vi "SpectroMeterConnectCheck.vi"(0 "error in":errorcluster) -> (1 "error Out":errorcluster caption="error out", 2 "LightField Automation out":refnum<class "LightField Automation.lvclass">)   [LabVIEW 2018]
uses:
  C:/ProgramData/Documents/Princeton Instruments/LightField/Add-in and Automation SDK/Samples/LabVIEW Automation/lightfield-automation-labview/LightField Automation.lvclass
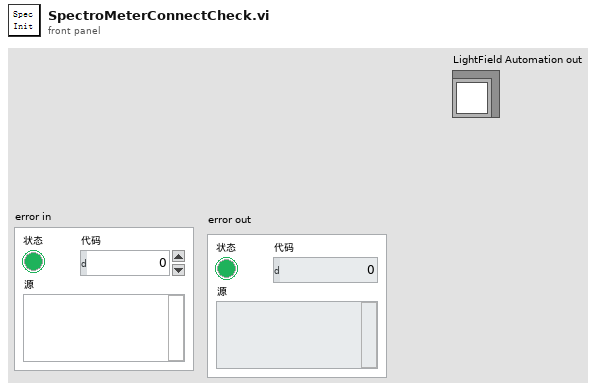
[diagram p1: front panel]
types:
  T1 = typedef "IMAQ Image.ctl" = refnum<image>
  T2 = cluster{"示波器":cluster{"Channel (0:Channel 1)":enum16{"Channel 1", "Channel 2", "Channel 3", "Channel 4"}, "电压范围":dbl, "触发电压":dbl, "时间范围":dbl, " 示波器VISA":refnum<visa-resource-name>, "时间范围 标签":u64, "电压范围 标签":u64, "触发电压 标签":u64, "输入阻抗/Ω":u64}, "光谱仪":cluster{"SpecDataReference":refnum<queue>, "grating center":dbl, "Exposure Time (s)":dbl, "是否进行详细设置":bool, " 开始通信检查":bool, "通信成功？":bool, "波长":dbl}, " 近场相机":cluster{"曝光时间/us":dbl, "模拟增益":i32, "控制套接字":i32, "IP 地址":string, " 采集套接字":i32, "  版本号":i32, "ImageData":T1, "  增益最大":i32, "  增益最小":i32, " 曝光最大":i32, " 曝光最小":i32, " 帧速":i32, " 同步切换":i32, "  曝光缩放":i32, "Camera Source":refnum<k21>, "近场X范围":dbl, "近场Y范围":dbl, "单个像元大小/um":dbl, "相机距离原点位置":dbl[]}, " 偏振仪":cluster{"电压范围":u64, "触发电压":u64, "时间范围":u64, "波长范围":enum16{"可见光 400-700nm", "近红外 700-1100nm"}, "可见光偏振测量仪VISA":refnum<visa-resource-name>, "近红外偏振测量仪VISA":refnum<visa-resource-name>}, " 功率计":cluster{"通道":enum16{"Channel 1", "Channel 2"}, "工作波长":u32, "单位":u64, "时间范围":u64, "IP地址":string, "端口":u32}, "能量计":cluster{"通道":enum16{"Channel 1", "Channel 2"}, "工作波长":u32, "单位":u64, "时间范围":u64, "IP地址":string, "端口":u32, "能量计量程":enum16{"200uJ", "20uJ", "2uJ", "200nJ"}}, "电机":cluster{"Channel (0:Channel 1)":enum16{"Channel 1", "Channel 2", "Channel 3", "Channel 4"}, "电压范围":u64, "触发电压":u64, "时间范围":u64}, " 远场相机":cluster{"曝光时间":i32, "模拟增益":i32, "控制套接字":i32, "IP 地址":string, " 采集套接字":i32, "  版本号":i32, "ImageData":T1, "  增益最大":i32, "  增益最小":i32, " 曝光最大":i32, " 曝光最小":i32, " 帧速":i32, " 同步切换":i32, "  曝光缩放":i32, "ImageData B":T1}}
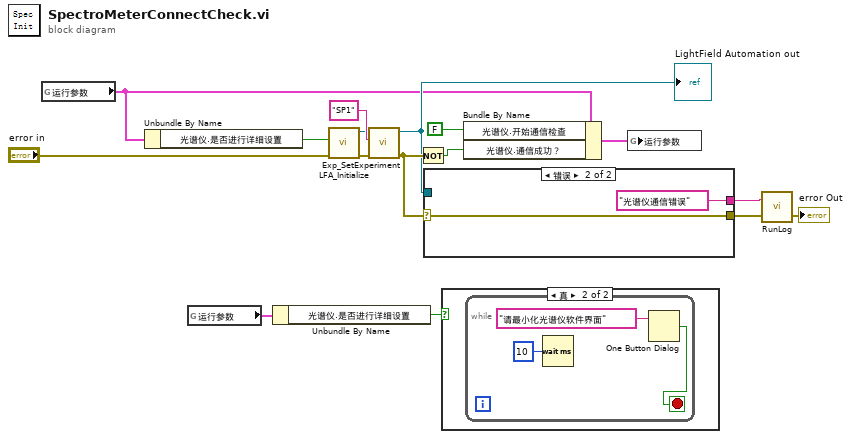
[diagram p0: block diagram]
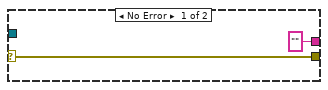
[diagram p3: hidden frame]
diagram:
  n1 = global read "参数.vi" "运行参数"() -> (w4:T2)
  n2 = Unbundle By Name(w4) -> ("光谱仪.是否进行详细设置"=w3:bool)
  n3 = global read "参数.vi" "运行参数"() -> (w2:T2)
  n4 = Unbundle By Name(w2) -> ("光谱仪.是否进行详细设置"=w1:bool)
  n5 = call "LFA_Initialize.vi"("error in (no error)"="error in", "Is Visible?"=w3) -> ("error out"=w9:errorcluster, "LightField Automation out"=w10:refnum<class "LightField Automation.lvclass">)  [unwired: 8 in]
  n6 = call "Exp_SetExperiment.vi"("error in (no error)"=w9, "ExperimentName"="SP1" ("Experiment Name"), "LightField Automation in"=w10) -> ("error out"=w13:errorcluster, "LightField Automation out"=w8:refnum<class "LightField Automation.lvclass">)  [unwired: 7 in]
  "LightField Automation out" <- w8
  n7 = Not(x=w13) -> (.not. x?=w6:bool)
  n8 = case shown="错误" w13 {
    selector: w13 -> [w18 w19]
    tunnel: [w18 w19] -> w12
    tunnel: w8 -> [_ _]
    tunnel: ["" "光谱仪通信错误" ("Message")] -> w15
    frame No Error {
    }
    frame Error {
    }
  }
  n9 = case shown="真" w1 {
    frame False {
    }
    frame True {
      n10 = while {
        stop <- w22 stop-if-true
        n11 = Wait (ms)(milliseconds to wait=u32 10 ("等待时间（毫秒）")) -> ()  [unwired: 1 out]
        n12 = One Button Dialog(message="请最小化光谱仪软件界面" ("消息")) -> (true=w22:bool)  [unwired: 1 in]
      }
    }
  }
  n13 = Bundle By Name(cluster=w4, "光谱仪.开始通信检查"=FALSE ("光谱仪. 开始通信检查"), "光谱仪.通信成功？"=w6) -> (w11:T2)
  n14 = global write "参数.vi" "运行参数"(w11) -> ()
  n15 = call "RunLog.vi"("error in"=w12, "Message"=w15) -> ("error out"=→"error Out":errorcluster)  [unwired: 1 in]
